vi "ZCAN_FilterClear.vi"(0 "error in (no error)":errorcluster caption="错误输入（无错误）", 2 "can_index_handle":u64) -> (14 "error out":errorcluster caption="错误输出", 16 "can_index_handle(out)":u64)   [LabVIEW 2018, in "zlgcan.lvlib"]
doc: "清除滤波表格"
uses:
  zlgcan.lvlib
  bin/ControlCANFD.dll
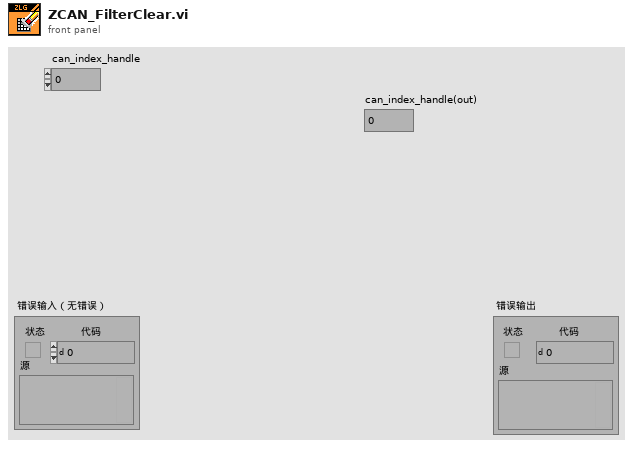
[diagram p1: front panel]
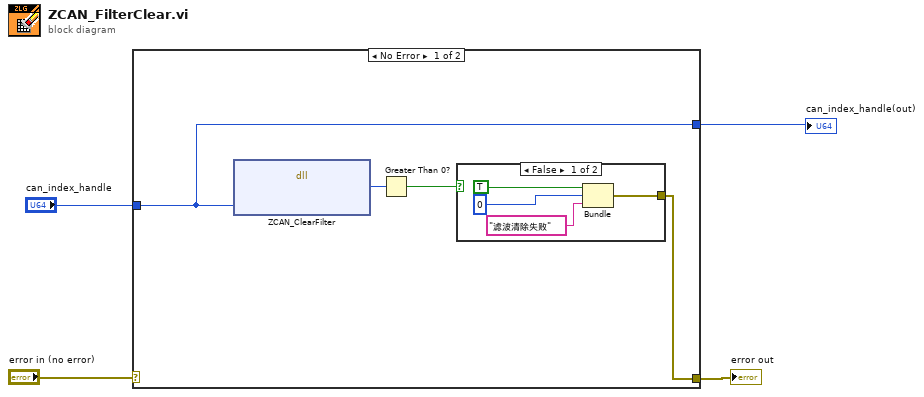
[diagram p0: block diagram]
diagram:
  n1 = case shown="No Error" "error in (no error)" {
    selector: "error in (no error)" -> [_ w13]
    tunnel: [w7 w13] -> w3
    tunnel: "can_index_handle" -> [w5 _]
    tunnel: [w5 _] -> w1
    frame No Error {
      n2 = dll-call lib="C:/Users/ttc52/Desktop/DHC FD LV2018/LABIVIEW CANFD Tool_V1.2.4_20220724/bin/ControlCANFD.dll" fn="ZCAN_ClearFilter"("device_handle"=w5) -> ("return"=w6:u32)  [unwired: 4 in, 2 out]
      n3 = Greater Than 0?(x=w6) -> (x > 0?=w8:bool)
      n4 = case shown="False" w8 {
        tunnel: [w9 _] -> w7
        frame False {
          n5 = Bundle("status"=TRUE, "code"=0, "消息"="滤波清除失败") -> (w9:cluster{"status":bool, "code":i32, "消息":string})  [unwired: 1 in]
        }
        frame True {
        }
      }
    }
    frame Error {
    }
  }
  "error out" <- w3
  "can_index_handle(out)" <- w1
